vi "Takeoff.vi"(11 "UDP Output Port":refnum<k16>) -> (3 "UDP Output Port 2":refnum<k16>)   [LabVIEW 2011]
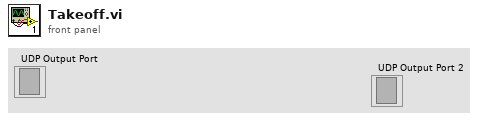
[diagram p1: front panel]
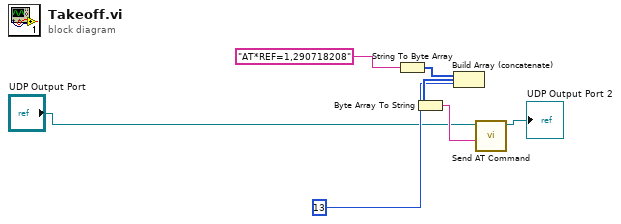
[diagram p0: block diagram]
diagram:
  n1 = String To Byte Array(string="AT*REF=1,290718208") -> (unsigned byte array=w6:u8[])
  n2 = Build Array (concatenate)(w6, u8 13) -> (w7:u8[])
  n3 = Byte Array To String(unsigned byte array=w7) -> (string=w4:string)
  n4 = call "Send AT Command.vi"("AT Command"=w4, "UDP Output Port"="UDP Output Port") -> ("UDP Output Port"=→"UDP Output Port 2":refnum<k16>)  [unwired: 9 in]
